vi "UDP Begin Packet URL Test.vi"() -> ()   [LabVIEW 2014, in "ESP8266 WiFi Wrapper.lvlib"]
uses:
  <vilib>/Aledyne-TSXperts/Arduino Compatible Compiler for LabVIEW/addons/ESP8266 WiFi Wrapper/ESP8266 WiFi Wrapper.lvlib
panel:
  in  "Port":i16=8266
  in  "Host Name":string="Example host name"
  out "Successful?":bool
  out "Error Out":errorcluster
  in  "Error In":errorcluster
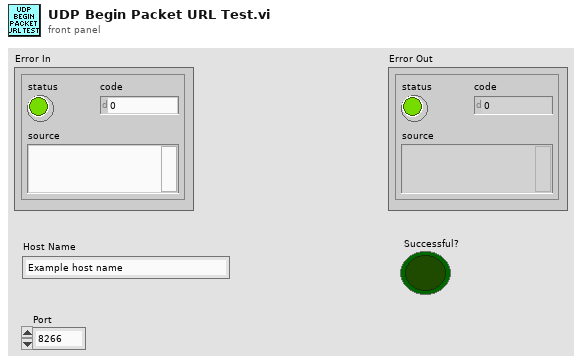
[diagram p1: front panel]
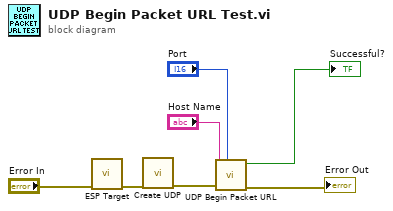
[diagram p0: block diagram]
diagram:
  n1 = call <vilib>:"ESP Target.vi"("Error In"="Error In") -> ("Error Out"=w6:errorcluster)  [unwired: 10 in]
  n2 = call <vilib>:"Create UDP.vi"("Error In"=w6) -> ("Error Out"=w5:errorcluster)  [unwired: 10 in]
  n3 = call <vilib>:"UDP Begin Packet URL.vi"("Port"="Port", "Error In"=w5, "Host Name"="Host Name") -> ("Error Out"=→"Error Out":errorcluster, "Successful?"=→"Successful?":bool)  [unwired: 7 in]
